vi "Setfocus_pointbypoint.vi"(0 "Z start (V)":dbl=5.180752688171838, 1 "time per point (s)":dbl=0.2 format="%#_6p", 2 "Z end (V)":dbl=5.580752688171838 format="%.2f", 3 "#steps":i32=40, 4 "set stage to zero before scan? (to avoid hysteresis)":bool=TRUE, 5 "counts_focus":refnum<vi>) -> (7 "Z max (V)":dbl=5.180752688171838)   [LabVIEW 2014]
uses:
  global_variables_AWG.vi
  global_channels.vi
panel:
  in  "stop":bool
  out "Z-position":dbl=5.380752688171838
  out "step size (V)":dbl=0.010000000000000009
  out "Z focus":cluster{dbl[], "histogram plot":dbl[]}(graph)={[5.180752688171838, 5.1907526881718375, 5.200752688171837, 5.210752688171837, 5.220752688171837, 5.230752688171837, 5.2407526881718365, 5.250752688171836, 5.260752688171836, 5.270752688171836, 5.280752688171836, 5.290752688171835, 5.300752688171835, 5.310752688171835, 5.320752688171835, 5.330752688171835, 5.340752688171834, 5.350752688171834, 5.360752688171834, 5.370752688171834, 5.3807526881718335, 5.390752688171833, 5.400752688171833, 5.410752688171833, 5.420752688171833, 5.430752688171832, 5.440752688171832, 5.450752688171832, 5.460752688171832, 5.470752688171832, 5.480752688171831, 5.490752688171831, 5.500752688171831, 5.510752688171831, 5.5207526881718305, 5.53075268817183, 5.54075268817183, 5.55075268817183, 5.56075268817183, 5.5707526881718294, 5.580752688171829], "histogram plot"=[23395.0, 17140.0, 16510.0, 17170.0, 17485.0, 17410.0, 18545.0, 18605.0, 22810.0, 20535.0, 20850.0, 20735.0, 20835.0, 19880.0, 20435.0, 21280.0, 20420.0, 19835.0, 20345.0, 20200.0, 19995.0, 18990.0, 19640.0, 18755.0, 18940.0, 19245.0, 17845.0, 18180.0, 17570.0, 18075.0, 17675.0, 18220.0, 17985.0, 19820.0, 18565.0, 17840.0, 18230.0, 18475.0, 17570.0, 18265.0, 17600.0]}
  # "Current Z"
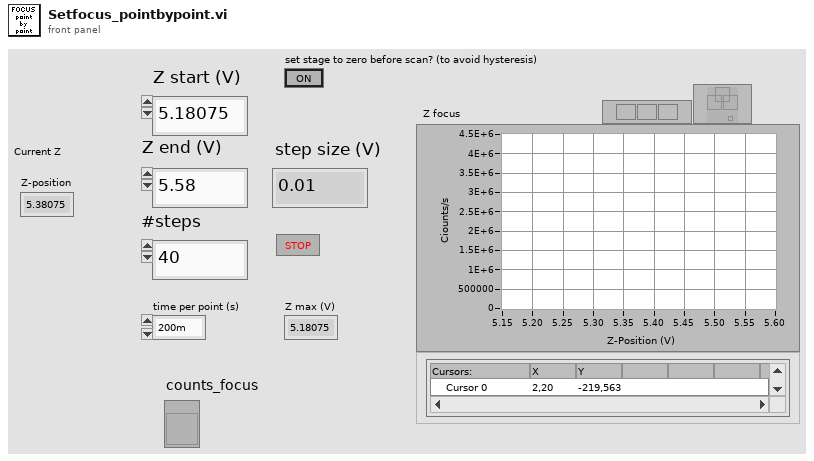
[diagram p1: front panel]
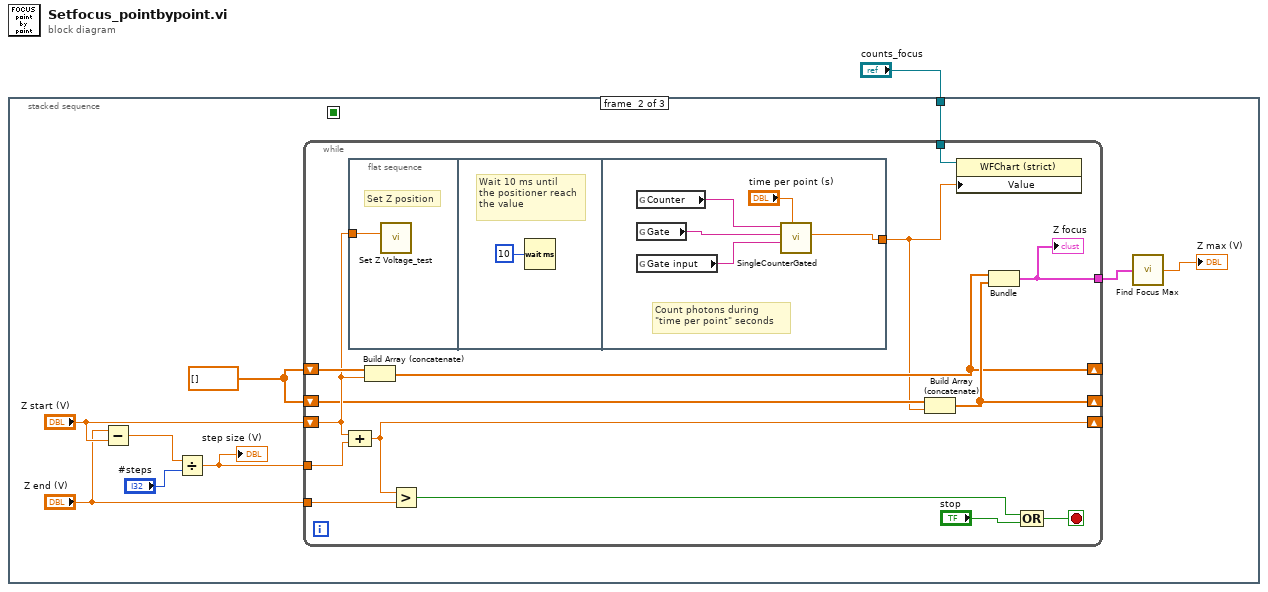
[diagram p0: block diagram]
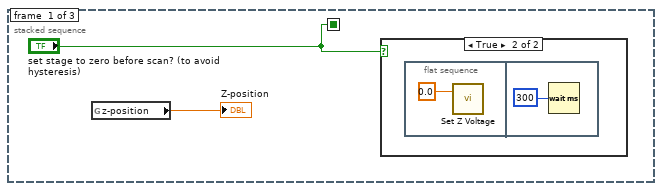
[diagram p2: hidden frame]
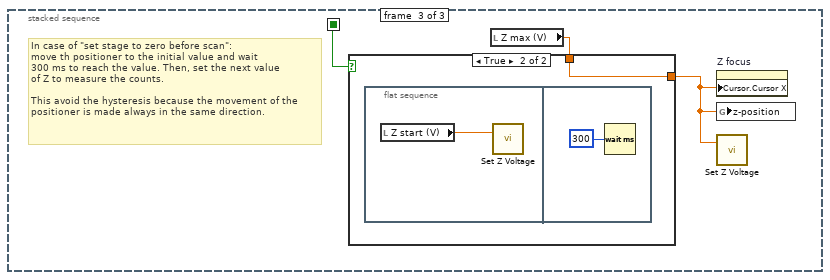
[diagram p4: hidden frame]
diagram:
  n1 = stacked-sequence {
    seq-local: ["set stage to zero before scan? (to avoid hysteresis)" _ _] -> [_ _ w38]
    tunnel: "counts_focus" -> [_ w6 _]
    frame #0 {
      n2 = global read "global_variables_AWG.vi" "z-position"() -> (→"Z-position":dbl)
      n3 = case shown="True" "set stage to zero before scan? (to avoid hysteresis)" {
        frame False {
        }
        frame True {
          n4 = flat-sequence {
            frame #0 {
              n5 = call "Set Z Voltage.vi"("Z position (V)"=0.0) -> ()  [unwired: 2 in]
            }
            frame #1 {
              n6 = Wait (ms)(milliseconds to wait=u32 300) -> ()  [unwired: 1 out]
            }
          }
        }
      }
    }
    frame #1 {
      w11 = dbl[] []
      n7 = Subtract(x="Z end (V)", y="Z start (V)") -> (x-y=w14:dbl)
      n8 = Divide(x=w14, y="#steps") -> (x/y=w12:dbl)
      "step size (V)" <- w12
      n9 = while {
        shift-right: [w27] -> _
        shift-left: "Z start (V)" -> [w21]
        tunnel: w12 -> [w28]
        tunnel: "Z end (V)" -> [w26]
        shift-right: [w18] -> _
        shift-left: w11 -> [w22]
        shift-right: [w19] -> _
        shift-left: w11 -> [w20]
        tunnel: [w16] -> w7
        tunnel: w6 -> [w17]
        stop <- w23 stop-if-true
        n10 = flat-sequence {
          tunnel: w21 -> [w29]
          tunnel: [w31] -> w15
          frame #0 {
            # "Set Z position"
            n11 = call "Set Z Voltage_test.vi"("Z-Position"=w29) -> ()  [unwired: 9 in]
          }
          frame #1 {
            # "Wait 10 ms until\nthe positioner reach\nthe value"
            n12 = Wait (ms)(milliseconds to wait=u32 10) -> ()  [unwired: 1 out]
          }
          frame #2 {
            # "Count photons during\n\"time per point\" seconds"
            n13 = global read "global_channels.vi" "Counter"() -> (w35:tag)
            n14 = global read "global_channels.vi" "Gate"() -> (w34:tag)
            n15 = global read "global_channels.vi" "Gate input"() -> (w33:tag)
            n16 = call "SingleCounterGated.vi"("Acquisition time [s]"="time per point (s)", "Gate input"=w33, "Gate"=w34, "Counter"=w35) -> ("counts/s"=w31:dbl)  [unwired: 5 in, 2 out]
          }
        }
        n17 = Compound Arithmetic op=ADD(w21, w28) -> (w27:dbl)
        n18 = Build Array (concatenate)(w22, w21) -> (w18:dbl[])
        n19 = Greater?(x=w27, y=w26) -> (0:w25:bool)
        n20 = Build Array (concatenate)(w20, w15) -> (w19:dbl[])
        n21 = property class="WFChart (strict)"(reference=w17, "Value"=w15) -> ()  [unwired: 1 in, 2 out]
        n22 = Bundle(w18, w19) -> (w16:cluster{dbl[], dbl[]})  [unwired: 1 in]
        "Z focus" <- w16
        n23 = Compound Arithmetic op=OR(w25, "stop") -> (w23:bool)
      }
      n24 = call "Find Focus Max.vi"("Averaged Ratio"=w7) -> ("Value of Z for max counts"=→"Z max (V)":dbl)  [unwired: 6 in]
    }
    frame #2 {
      # "In case of \"set stage to zero before scan\":\nmove th positioner to the initial value and wait\n300 ms to reach the value. Then, set the next value\nof Z to measure the counts.\n\nThis avoid the hysteresis because the movement of the\npositioner is made always in the same direction."
      n25 = local read "Z max (V)"() -> (w37:dbl)
      n26 = case shown="True" w38 {
        tunnel: [w39 w40] -> w36
        tunnel: w37 -> [w39 w40]
        frame False {
        }
        frame True {
          n27 = flat-sequence {
            frame #0 {
              n28 = local read "Z start (V)"() -> (w41:dbl)
              n29 = call "Set Z Voltage.vi"("Z position (V)"=w41) -> ()  [unwired: 2 in]
            }
            frame #1 {
              n30 = Wait (ms)(milliseconds to wait=u32 300) -> ()  [unwired: 1 out]
            }
          }
        }
      }
      n31 = property on="Z focus" class="XYGraph (strict)"("Cursor.Cursor X"=w36) -> ()  [unwired: 2 in, 2 out]
      n32 = global write "global_variables_AWG.vi" "z-position"(w36) -> ()
      n33 = call "Set Z Voltage.vi"("Z position (V)"=w36) -> ()  [unwired: 2 in]
    }
  }
